vi "Read Input String.vi"(0 "Input":string) -> (7 "Msg Out":string, 8 "Nu":dbl[](array[numeric]), 9 "Eta":dbl[](array[numeric]), 10 "Nu_est":dbl[](array[numeric]), 11 "Eta_d":dbl[](array[numeric]), 12 "Nu_d":dbl[](array[numeric]), 13 "Array":bool[](array[boolean])=[TRUE], 14 "Des Depth [m]":dbl, 15 "Depth [m]":dbl, 17 "Heading [deg]":dbl, 18 "Des Heading [deg]":dbl, 19 "Eta_est":dbl[](array[numeric]))   [LabVIEW 2014]
panel:
  out "error out":errorcluster
  in  "error in":errorcluster
  out "Cluster Position":cluster{"Pos North":dbl, "Pos East":dbl}
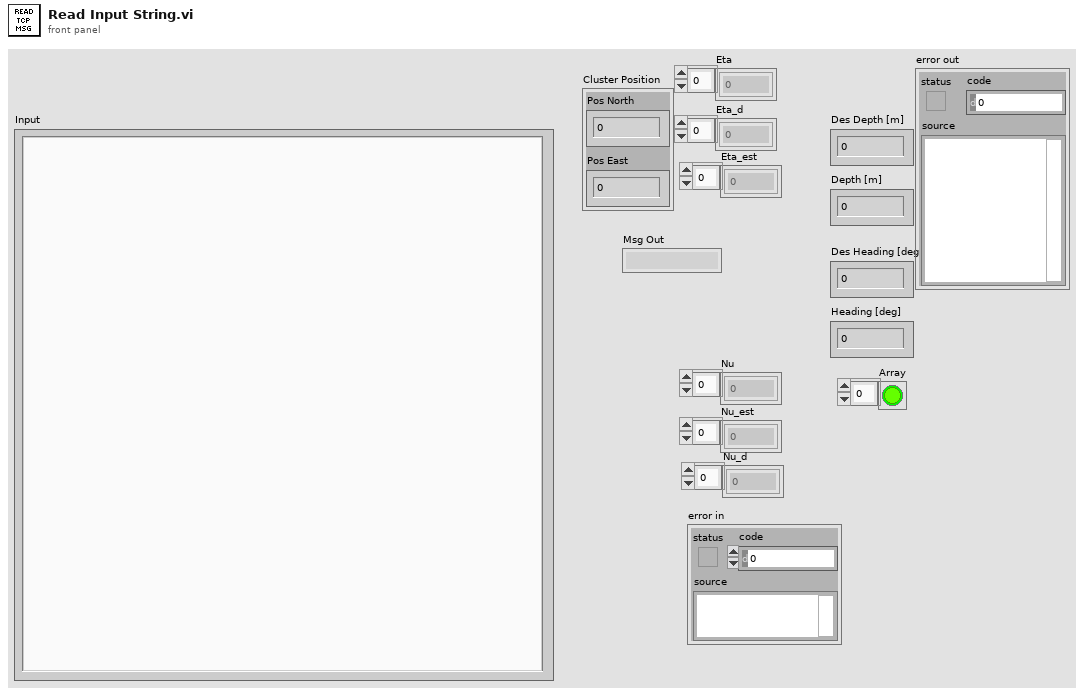
[diagram p1: front panel]
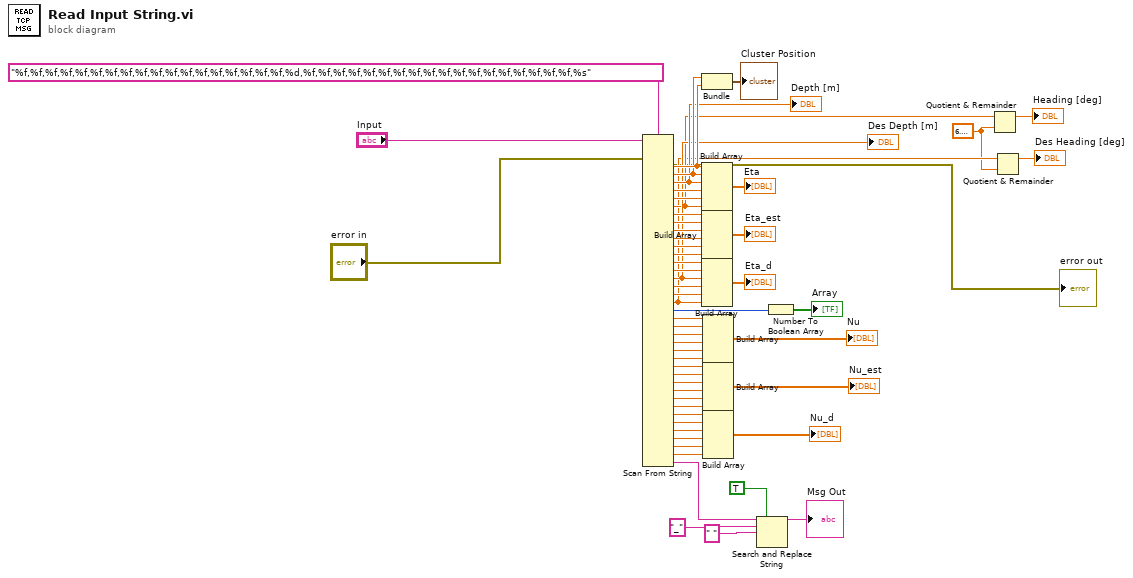
[diagram p0: block diagram]
diagram:
  w13 = 6.283185307179586
  n1 = Scan From String(format string="%f,%f,%f,%f,%f,%f,%f,%f,%f,%f,%f,%f,%f,%f,%f,%f,%f,%f,%d,%f,%f,%f,%f,%f,%f,%f,%f,%f,%f,%f,%f,%f,%f,%f,%f,%f,%f,%s", input string="Input", error in="error in") -> (error out=→"error out":errorcluster, output 1=w41:dbl, output 2=w40:dbl, output 3=w39:dbl, output 4=w47:dbl, output 5=w46:dbl, output 6=w15:dbl, output 7=w45:dbl, output 8=w44:dbl, output 9=w38:dbl, output 10=w43:dbl, output 11=w42:dbl, output 12=w37:dbl, output 13=w35:dbl, output 14=w34:dbl, output 15=w16:dbl, output 16=w33:dbl, output 17=w32:dbl, output 18=w14:dbl, output 19=w31:i32, output 20=w30:dbl, output 21=w29:dbl, output 22=w28:dbl, output 23=w27:dbl, output 24=w26:dbl, output 25=w25:dbl, output 26=w24:dbl, output 27=w23:dbl, output 28=w22:dbl, output 29=w21:dbl, output 30=w20:dbl, output 31=w19:dbl, output 32=w10:dbl, output 33=w9:dbl, output 34=w8:dbl, output 35=w7:dbl, output 36=w6:dbl, output 37=w5:dbl, output 38=w4:string)  [unwired: 39 in, 2 out]
  "Des Depth [m]" <- w16
  "Depth [m]" <- w39
  n2 = Bundle(w40, w41) -> (→"Cluster Position":cluster{dbl, dbl})  [unwired: 1 in]
  n3 = Build Array(w41, w40, w39, w47, w46, w15) -> (→"Eta":dbl[])
  n4 = Build Array(w45, w44, w38, w43, w42, w37) -> (→"Eta_est":dbl[])
  n5 = Build Array(w35, w34, w16, w33, w32, w14) -> (→"Eta_d":dbl[])
  n6 = Build Array(w30, w29, w28, w27, w26, w25) -> (→"Nu":dbl[])
  n7 = Build Array(w24, w23, w22, w21, w20, w19) -> (→"Nu_est":dbl[])
  n8 = Build Array(w10, w9, w8, w7, w6, w5) -> (→"Nu_d":dbl[])
  n9 = Search and Replace String(replace all?=TRUE, input string=w4, search string="_", replace string=" ") -> (result string=→"Msg Out":string)  [unwired: 4 in, 3 out]
  n10 = Number To Boolean Array(number=w31) -> (Boolean array=→"Array":bool[])
  n11 = Quotient & Remainder(x=w15, y=w13) -> (x-y*floor(x/y)=→"Heading [deg]":dbl)  [unwired: 1 out]
  n12 = Quotient & Remainder(x=w14, y=w13) -> (x-y*floor(x/y)=→"Des Heading [deg]":dbl)  [unwired: 1 out]
